vi "Start Module.vi"(6 "Show Main VI Diagram on Init (F)":bool, 8 "error in":errorcluster) -> (0 "error out":errorcluster, 1 "Wait for Event Sync?":bool, 2 "My Singleton Module Broadcast Events":T1, 3 "Module Was Already Running?":bool, 4 "Module Name":string)   [LabVIEW 2020, in "My Singleton Module.lvlib"]
doc: "Launches the module Main VI. After calling this VI, you can optionally register for broadcast events from the module by wiring the broadcast events output of this VI to a <b>Register For Events</b> function. \n\nAfter the optional Register For Events function call, you should always call the <b>Synchronize Module Events.vi</b> for this module with the 'Wait for Event Sync?' output of this VI to the corresponding input of the Synchronize Module Events.vi. \n\nTo see an example of the proper wiring pattern, see the \"Start Module: Value Change\" event frame in the API Tester VI for this module.\n\nThe <b>Validate DQMH Module</b> tool added a 'Module Name' output to this VI.\n_____\nBased on DQMH Dev Tools: Project Template 7.1.0.1499."
uses:
  My Singleton Module.lvlib
  Broadcast Events--cluster.ctl
  Did Init Argument--cluster.ctl
  Status Updated Argument--cluster.ctl
  Error Reported Argument--cluster.ctl
  Do Something Argument--cluster.ctl
  Stop Argument--cluster.ctl
  Get Module Execution Status Argument--cluster.ctl
  <vilib>/Delacor/Delacor QMH/Libraries/Module Admin_class/Delacor_lib_QMH_Module Admin.lvclass
  <vilib>/Delacor/Delacor QMH/Libraries/Module Admin_class/Delacor_lib_QMH_Module Admin.lvclass/Delacor_lib_QMH_Module Admin.ctl
  <vilib>/Delacor/Delacor QMH/Libraries/Module Admin_class/Delacor_lib_QMH_Set External Launch.vi
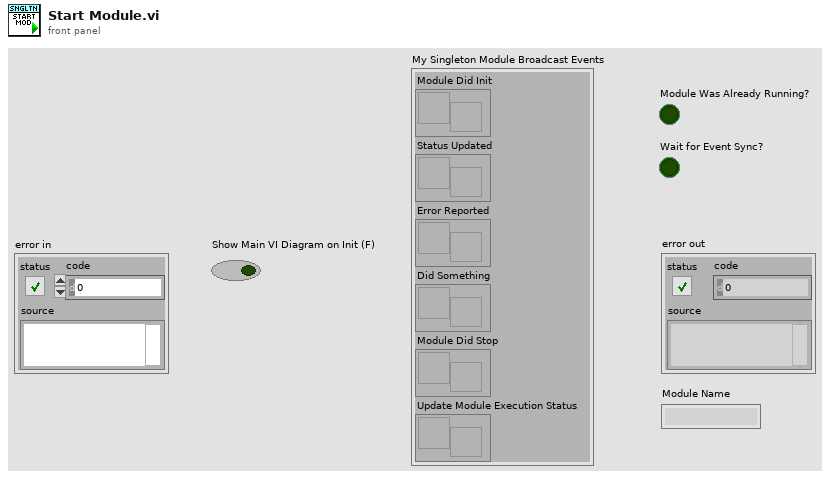
[diagram p1: front panel]
types:
  T1 = typedef "My Singleton Module.lvlib/Broadcast Events--cluster.ctl" = cluster{"Module Did Init":refnum<user-event>, "Status Updated":refnum<user-event>, "Error Reported":refnum<user-event>, "Did Something":refnum<user-event>, "Module Did Stop":refnum<user-event>, "Update Module Execution Status":refnum<user-event>}
  T2 = enum32{"Bad", "Idle", "Run top level", "Running"}
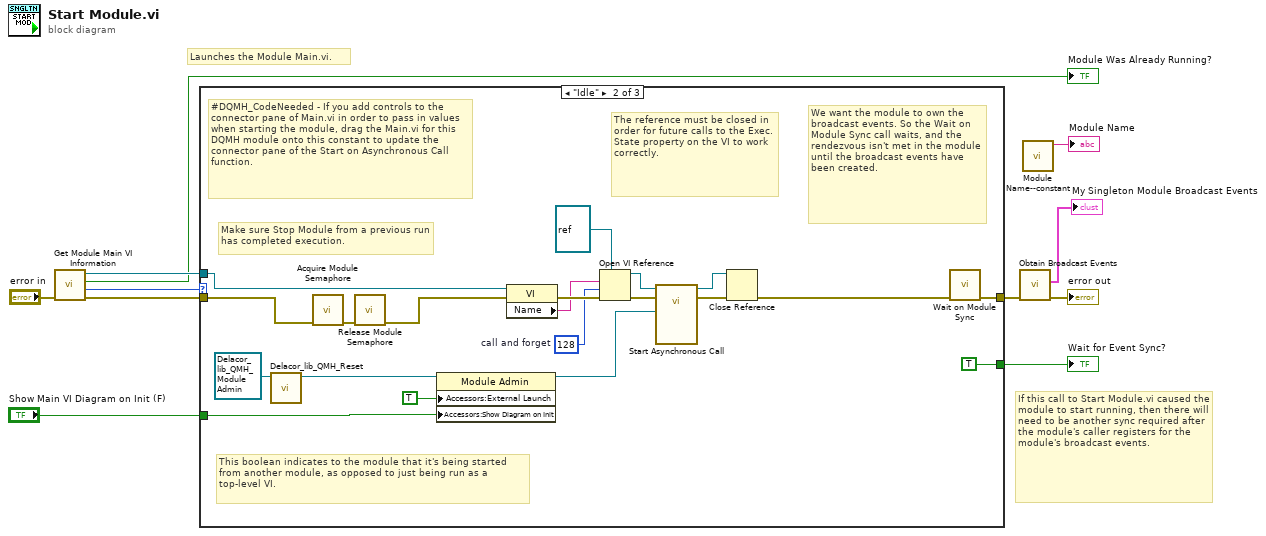
[diagram p0: block diagram]
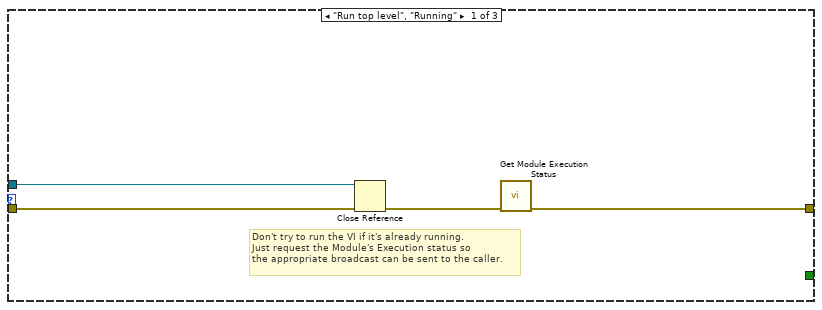
[diagram p2: hidden frame]
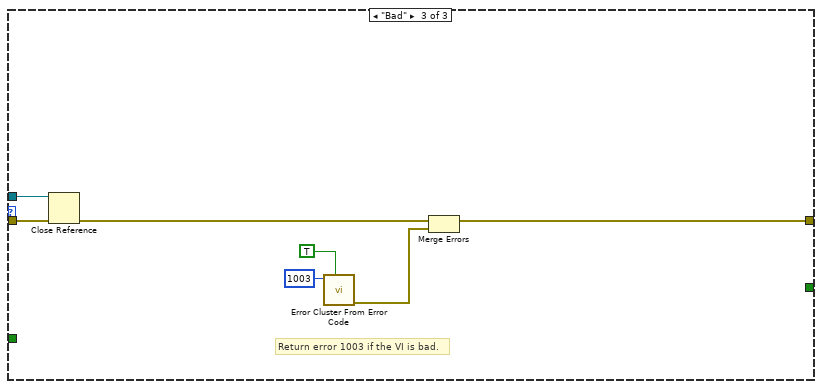
[diagram p3: hidden frame]
diagram:
  # "If this call to Start Module.vi caused the module to start running, then there will need to be another sync required after the module's caller registers for the module's broadcast events."
  # "Launches the Module Main.vi."
  n1 = call "Get Module Main VI Information.vi"("error in"="error in") -> ("error out"=w11:errorcluster, "Execution State"=w6:T2, "Is Module Running?"=→"Module Was Already Running?":bool, "Module Main VI"=w10:refnum<vi>)  [unwired: 7 in]
  n2 = case shown="\"Idle\"" w6 {
    tunnel: w11 -> [w15 w18 w42]
    tunnel: w10 -> [w14 w30 w41]
    tunnel: [w12 w35 w39] -> w9
    tunnel: [_ TRUE _] -> w7
    tunnel: "Show Main VI Diagram on Init (F)" -> [_ w16 _]
    frame "Run top level", "Running" {
      # "Don't try to run the VI if it's already running.\nJust request the Module's Execution status so\nthe appropriate broadcast can be sent to the caller."
      n3 = Close Reference(reference=w14, error in (no error)=w15) -> (error out=w13:errorcluster)
      n4 = call "Get Module Execution Status.vi"("error in"=w13) -> ("error out"=w12:errorcluster)  [unwired: 10 in]
    }
    frame "Idle" {
      w27 = 128  # call and forget
      # "Make sure Stop Module from a previous run has completed execution."
      # "#DQMH_CodeNeeded - If you add controls to the connector pane of Main.vi in order to pass in values when starting the module, drag the Main.vi for this DQMH module onto this constant to update the connector pane of the Start on Asynchronous Call function."
      # "The reference must be closed in order for future calls to the Exec.State property on the VI to work correctly."
      # "We want the module to own the broadcast events. So the Wait on Module Sync call waits, and the rendezvous isn't met in the module until the broadcast events have been created."
      # "This boolean indicates to the module that it's being started from another module, as opposed to just being run as a top-level VI."
      n5 = call-dynamic "Delacor_lib_QMH_Reset.vi"("Mod Admin in"=refnum<class "Delacor_lib_QMH_Module Admin.lvclass"> refnum) -> ("Mod Admin out"=w33:refnum<class "Delacor_lib_QMH_Module Admin.lvclass">)  [unwired: 9 in, 1 out]
      n6 = call "Acquire Module Semaphore.vi"("error in"=w18) -> ("error out"=w19:errorcluster)  [unwired: 10 in]
      n7 = call "Release Module Semaphore.vi"("error in"=w19) -> ("error out"=w17:errorcluster)  [unwired: 10 in]
      n8 = property class="Module Admin"(reference=w33, "Accessors:External Launch"=TRUE, "Accessors:Show Diagram on Init"=w16) -> (reference out=w24:refnum<class "Delacor_lib_QMH_Module Admin.lvclass">)  [unwired: 1 in, 1 out]
      n9 = property class="VI"(reference=w30, error in=w17) -> (error out=w29:errorcluster, "Name"=w20:string)  [unwired: 1 out]
      n10 = Open VI Reference(type specifier VI Refnum (for type only)=refnum<vi> refnum, vi path=w20, options=w27, error in (no error)=w29) -> (vi reference=w25:refnum<vi>, error out=w26:errorcluster)  [unwired: 2 in]
      n11 = call-by-ref "Start Asynchronous Call"(reference=w25, error in=w26, "Module Admin"=w24) -> (reference out=w22:refnum<vi>, error out=w23:errorcluster)  [unwired: 11 in]
      n12 = Close Reference(reference=w22, error in (no error)=w23) -> (error out=w21:errorcluster)
      n13 = call "Wait on Module Sync.vi"("error in"=w21) -> ("error out"=w35:errorcluster)  [unwired: 10 in]
    }
    frame "Bad" {
      # "Return error 1003 if the VI is bad."
      n14 = Close Reference(reference=w41, error in (no error)=w42) -> (error out=w40:errorcluster)
      n15 = call <vilib>:"Error Cluster From Error Code.vi"("show call chain? (False)"=TRUE, "error code (0)"=1003) -> ("error out"=w38:errorcluster)  [unwired: 7 in]
      n16 = Merge Errors(w40, w38) -> (w39:errorcluster)
    }
  }
  "Wait for Event Sync?" <- w7
  n17 = call "Obtain Broadcast Events.vi"("error in"=w9) -> ("error out"=→"error out":errorcluster, "My Singleton Module Broadcast Events"=→"My Singleton Module Broadcast Events":T1)  [unwired: 9 in]
  n18 = call "Module Name--constant.vi"() -> ("Module Name"=→"Module Name":string)  [unwired: 11 in]
